vi "IMS Stepper Move.vi"(0 "Instrument Address":refnum<visa-resource-name>, 1 "Motor Number":u32=1 min=1 max=255 step=1, 2 "Distance":dbl=1.0 min=-193273528.32 max=193273528.0 step=0.09 format="%.2f", 3 "error in (no error)":errorcluster, 4 "Mode":bool) -> (5 "error out":errorcluster)   [LabVIEW 2018]
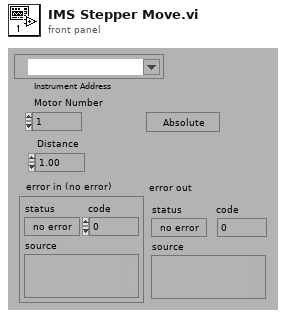
[diagram p1: front panel]
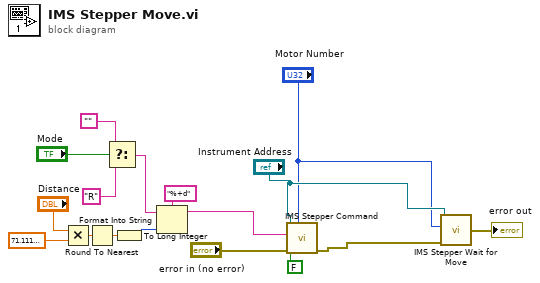
[diagram p0: block diagram]
diagram:
  n1 = Multiply(x="Distance", y=71.11111111) -> (x*y=w15:dbl)
  n2 = Round To Nearest(number=w15) -> (nearest integer value=w13:dbl)
  n3 = Select(t="", s="Mode", f="R") -> (s? t:f=w4:string)
  n4 = To Long Integer(number=w13) -> (32bit integer=w14:i32)
  n5 = Format Into String(format string="%+d", initial string=w4, w14) -> (resulting string=w3:string)  [unwired: 1 in, 1 out]
  n6 = call "IMS Stepper Command.vi"("Instrument Address"="Instrument Address", "Motor Number"="Motor Number", "Command"=w3, "Mode"=FALSE, "error in (no error)"="error in (no error)") -> ("error out"=w10:errorcluster)  [unwired: 1 in, 2 out]
  n7 = call "IMS Stepper Wait for Move.vi"("Instrument Address"="Instrument Address", "Motor Number"="Motor Number", "error in (no error)"=w10) -> ("error out"=→"error out":errorcluster)  [unwired: 2 in]
